vi "DigitalWatch.vi"() -> ()   [LabVIEW 2021]
panel:
  out "Mins":i32
  out "Secs":i32
  out "Hr":i32
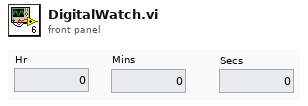
[diagram p1: front panel]
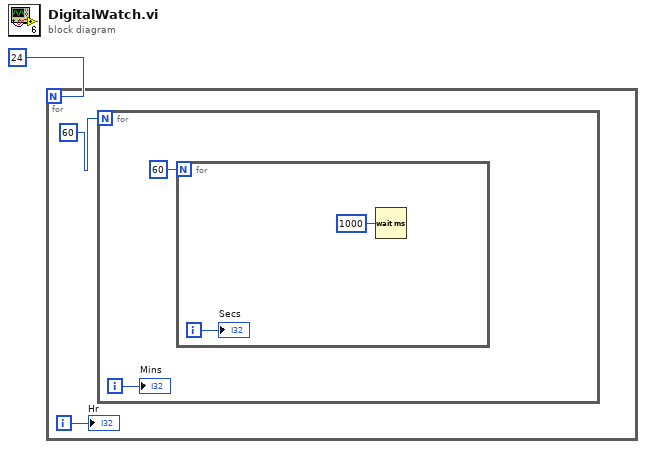
[diagram p0: block diagram]
diagram:
  n1 = for {
    N: 24 -> [_]
    i -> [w2]
    n2 = for {
      N: 60 -> [_]
      i -> [w4]
      n3 = for {
        N: 60 -> [_]
        i -> [w7]
        n4 = Wait (ms)(milliseconds to wait=u32 1000) -> ()  [unwired: 1 out]
        "Secs" <- w7
      }
      "Mins" <- w4
    }
    "Hr" <- w2
  }
